vi "dvm Config Panel.vi"(8 "error in (no error)":errorcluster, 11 "dvm session":T2) -> (0 "error out":errorcluster, 3 "dvm session out":T2)   [LabVIEW 2020]
doc: "Auxiliary DVM config panel."
uses:
  dvm session.ctl
  dvm type.ctl
  drivers/Fluke 5790A/top_level/F5790 session.ctl
panel:
  in  "btn cfg adc":bool
  in  "btn ok":bool
  in  "dvm type":T1 caption="DVM type"
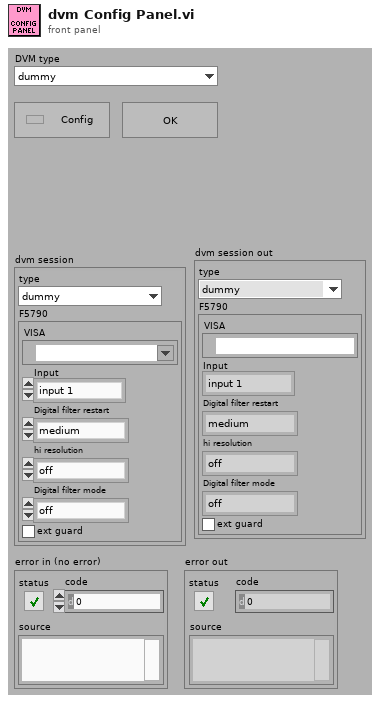
[diagram p1: front panel]
types:
  T1 = typedef "dvm type.ctl" = enum16{"dummy", "Fluke 5790A"}
  T2 = typedef "dvm session.ctl" = cluster{"type":T1, "F5790":T3}
  T3 = typedef "F5790 session.ctl" = cluster{"VISA":refnum<visa-resource-name>, "Input":enum16{"input 1", "input 2", "wide-band"}, "Digital filter restart":enum16{"medium", "fine", "coarse"}, "hi resolution":enum16{"off", "on"}, "Digital filter mode":enum16{"off", "fast", "medium", "slow"}, "ext guard":bool}
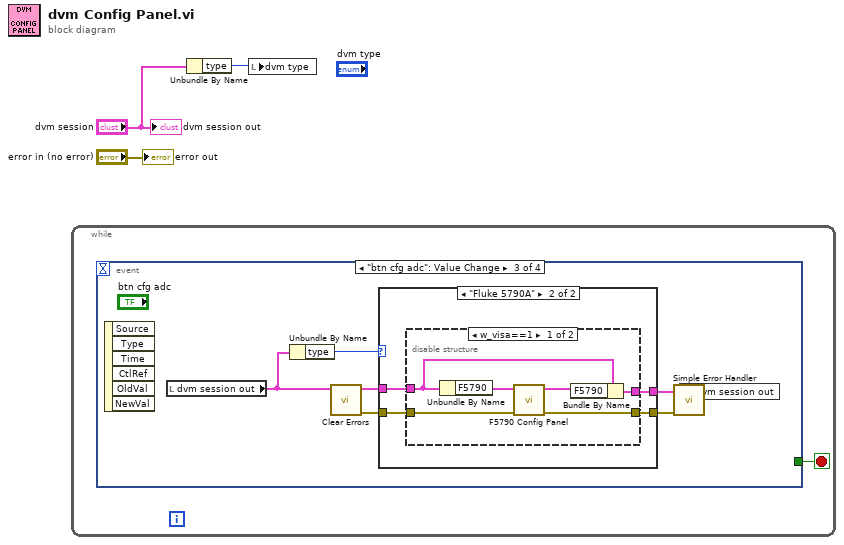
[diagram p0: block diagram]
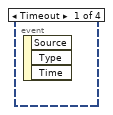
[diagram p2: hidden frame]
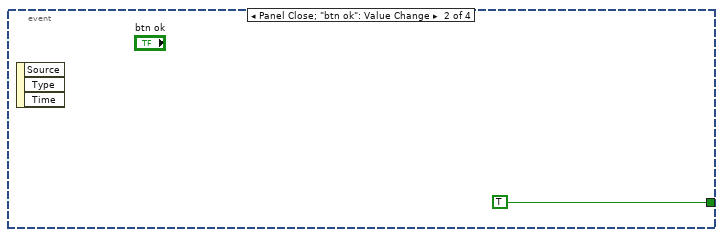
[diagram p3: hidden frame]
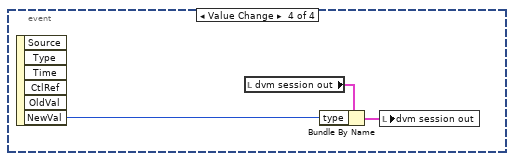
[diagram p6: hidden frame]
diagram:
  n1 = while {
    stop <- w4 stop-if-true
    n2 = event shown="[2] \"btn cfg adc\": Value Change" {
      selector: _ -> [_ _ _ _]
      dyn-events: _ -> [_ _ _ _]
      timeout: _ -> [_ _ _ _]
      tunnel: [_ TRUE _ _] -> w4
      event Timeout {
        n3 = event-data() -> ()  [unwired: 1 in, 3 out]
      }
      event Panel Close; "btn ok": Value Change {
        n4 = event-data() -> ()  [unwired: 1 in, 3 out]
      }
      event "btn cfg adc": Value Change {
        n5 = event-data() -> ()  [unwired: 1 in, 6 out]
        n6 = local read "dvm session out"() -> (w7:T2)
        n7 = Unbundle By Name(w7) -> ("type"=w6:T1)
        n8 = call <vilib>:"Clear Errors.vi"() -> ("error out"=w9:errorcluster)  [unwired: 6 in, 1 out]
        n9 = case shown="\"Fluke 5790A\"" w6 {
          tunnel: w9 -> [w12 w16]
          tunnel: [w12 w15] -> w10
          tunnel: w7 -> [w11 w14]
          tunnel: [w11 w13] -> w8
          frame "dummy", Default {
          }
          frame "Fluke 5790A" {
            n10 = disable-structure shown="w_visa==1" {
              disable-tunnel: w16 -> [w22 w24]
              disable-tunnel: [w21 w24] -> w15
              disable-tunnel: w14 -> [w19 w23]
              disable-tunnel: [w17 w23] -> w13
              frame condition #0 (active) {
                n11 = Unbundle By Name(w19) -> ("F5790"=w20:T3)
                n12 = call "F5790 Config Panel.vi"("error in (no error)"=w22, "F5790 session in"=w20) -> ("error out"=w21:errorcluster, "F5790 session out"=w18:T3)  [unwired: 8 in]
                n13 = Bundle By Name(cluster=w19, "F5790"=w18) -> (w17:T2)
              }
              frame condition #1 {
              }
            }
          }
        }
        n14 = call <vilib>:"Simple Error Handler.vi"("error in (no error)"=w10) -> ()  [unwired: 4 in, 5 out]
        n15 = local write "dvm session out"(w8) -> ()
      }
      event Value Change {
        n16 = event-data() -> ("NewVal"=w25:T1)  [unwired: 1 in, 5 out]
        n17 = local read "dvm session out"() -> (w27:T2)
        n18 = Bundle By Name(cluster=w27, "type"=w25) -> (w26:T2)
        n19 = local write "dvm session out"(w26) -> ()
      }
    }
  }
  n20 = Unbundle By Name("dvm session") -> ("type"=w1:T1)
  n21 = local write "dvm type"(w1) -> ()
  "error out" <- "error in (no error)"
  "dvm session out" <- "dvm session"
